vi "Plot scale refnum to LUT name.vi"(3 "Scale reference":refnum<vi>) -> (1 "scale reference variant lookup name":string)   [LabVIEW 2021, in "RocketPlot.lvlib"]
uses:
  RocketPlot.lvlib
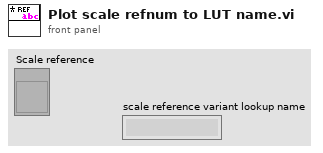
[diagram p1: front panel]
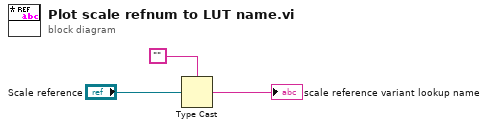
[diagram p0: block diagram]
diagram:
  n1 = Type Cast(type="", x="Scale reference") -> (*(type *) &x=→"scale reference variant lookup name":string)
